vi "safe_move_test.vi"() -> ()   [LabVIEW 2019]
uses:
  gVision/gVision.lvlib
panel:
  in  "end_label":string="needle_calibration_camera "
  in  "start_label":string="home"
  out "error out":errorcluster
  out "coordinates":cluster{"x":dbl, "y":dbl, "z":dbl}[](array[cluster])
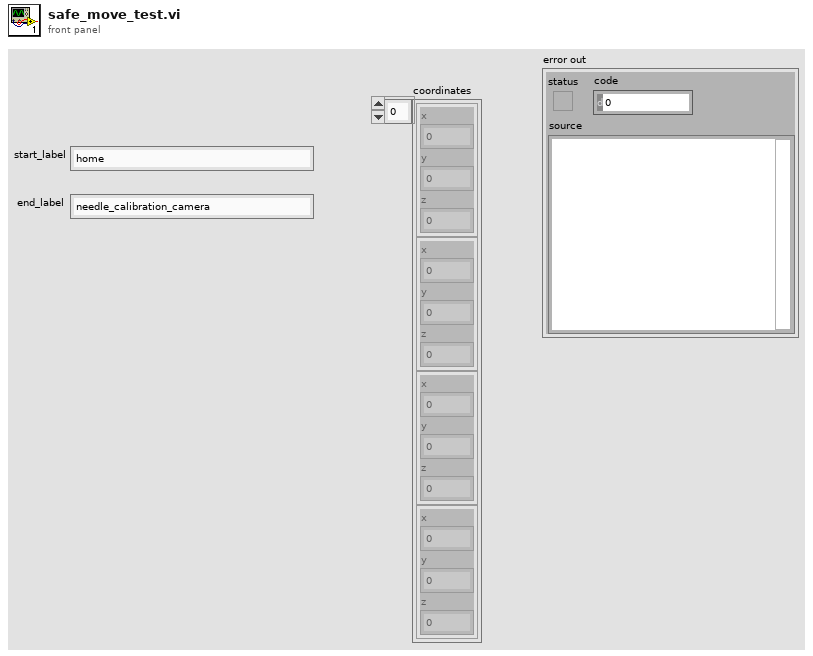
[diagram p1: front panel]
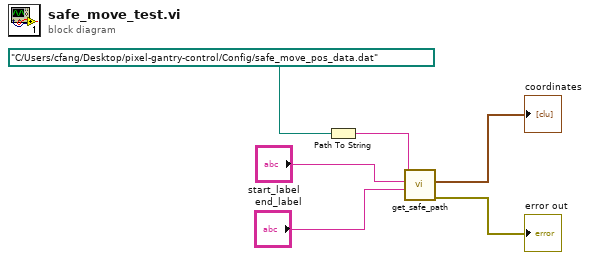
[diagram p0: block diagram]
diagram:
  n1 = Path To String(path=path "C:/Users/cfang/Desktop/pixel-gantry-control/Config/safe_move_pos_data.dat") -> (string=w5:string)
  n2 = call "get_safe_path.vi"("end_label"="end_label", "start_label"="start_label", "filename"=w5) -> ("error out"=→"error out":errorcluster, "coordinates"=→"coordinates":cluster{"x":dbl, "y":dbl, "z":dbl}[])  [unwired: 7 in]
